vi "Client_largefile.vi"() -> ()   [LabVIEW 2016, in "Sending_larger_data.lvlib"]
uses:
  Sending_larger_data.lvlib
  <vilib>/addons/zeromq/socket_type.ctl
  <vilib>/addons/zeromq/zmq_context.lvclass
  <vilib>/addons/zeromq/zeromq.lvlib
  <vilib>/addons/zeromq/zmq_socket.lvclass
panel:
  out "Power Spectrum":dbl[](graph)
  in  "cycles":dbl=500.0 format="%#_13g"
  in  "samples":i32=5000
  in  "Send":bool
  out "reply":string[](array[string])
  out "loop":string
  out "attempt":i32
  in  "stop":bool
  in  "ntries":i32=20
  in  "endpoint":string="tcp://127.0.0.1:5555"
  in  "timeout":u32=100
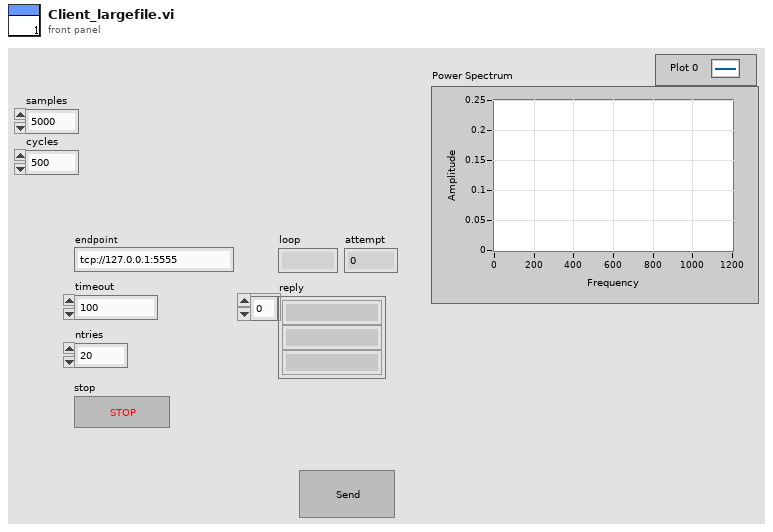
[diagram p1: front panel]
types:
  T1 = typedef "zeromq.lvlib/socket_type.ctl" = enum8{"ZMQ_PAIR", "ZMQ_PUB", "ZMQ_SUB", "ZMQ_REQ", "ZMQ_REP", "ZMQ_DEALER", "ZMQ_ROUTER", "ZMQ_PULL", "ZMQ_PUSH", "ZMQ_XPUB", "ZMQ_XSUB"}
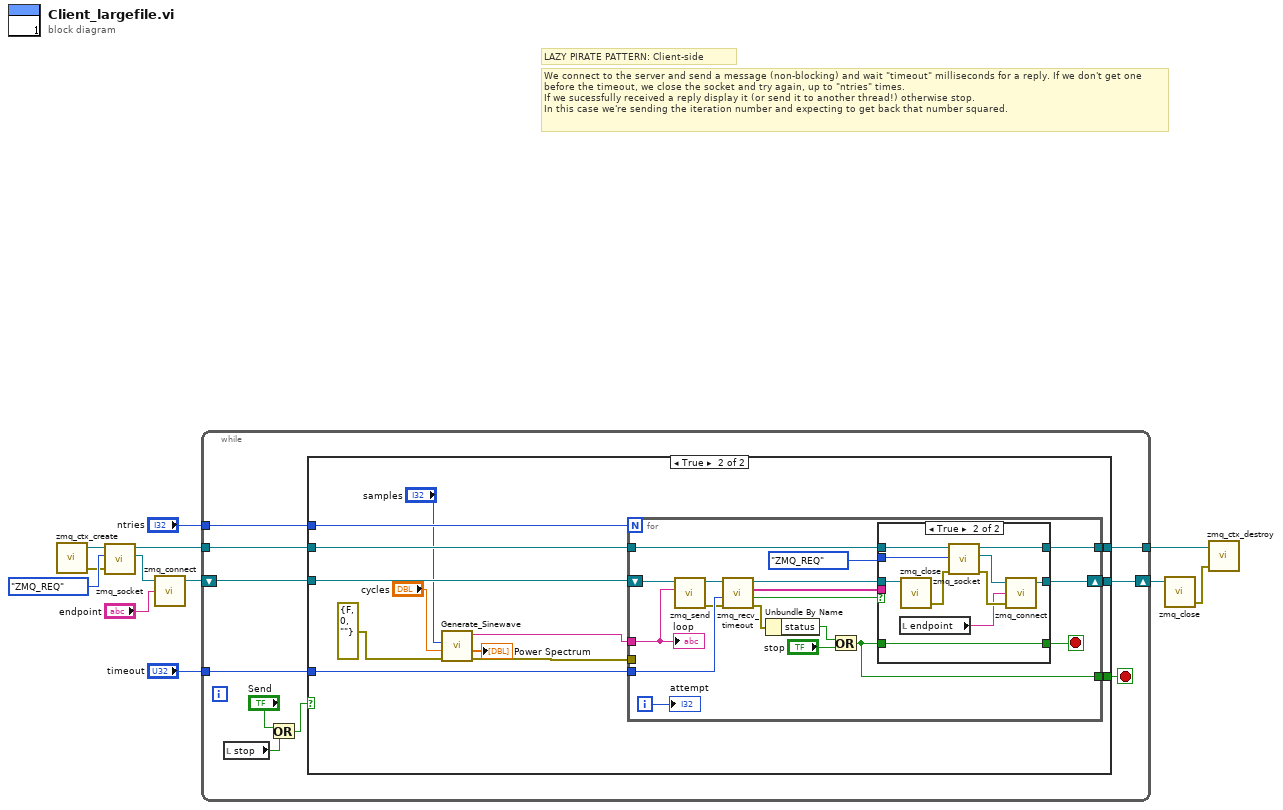
[diagram p0: block diagram]
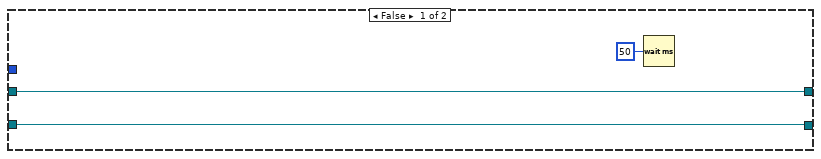
[diagram p2: hidden frame]
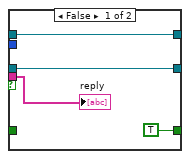
[diagram p3: hidden frame]
diagram:
  # "We connect to the server and send a message (non-blocking) and wait \"timeout\" milliseconds for a reply. If we don't get one before the timeout, we close the socket and try again, up to \"ntries\" times.\nIf we sucessfully received a reply display it (or send it to another thread!) otherwise stop.\nIn this case we're sending the iteration number and expecting to get back that number squared."
  # "LAZY PIRATE PATTERN: Client-side"
  n1 = call <vilib>:"zmq_ctx_create.vi"() -> ("error out"=w1:errorcluster, "context out"=w10:refnum<class "zmq_context.lvclass">)  [unwired: 4 in]
  n2 = call <vilib>:"zmq_socket.vi"("error in"=w1, "socket type"=socket_type."ZMQ_REQ", "context in"=w10) -> ("socket out"=w8:refnum<class "zmq_socket.lvclass">, "context out"=w7:refnum<class "zmq_context.lvclass">)  [unwired: 2 in, 1 out]
  n3 = call <vilib>:"zmq_connect.vi"("endpoint"="endpoint", "socket in"=w8) -> ("socket out"=w5:refnum<class "zmq_socket.lvclass">)  [unwired: 2 in, 1 out]
  n4 = while {
    tunnel: w7 -> [w22]
    tunnel: "timeout" -> [w21]
    tunnel: "ntries" -> [w20]
    tunnel: [w17] -> w4
    shift-right: [w16] -> w3
    shift-left: w5 -> [w18]
    stop <- w19 stop-if-true
    n5 = local read "stop"() -> (w14:bool)
    n6 = Or(x="Send", y=w14) -> (x .or. y?=w13:bool)
    n7 = case shown="True" w13 {
      tunnel: w22 -> [w24 w38]
      tunnel: w21 -> [_ w37]
      tunnel: w20 -> [_ w36]
      tunnel: [_ w35] -> w19
      tunnel: w18 -> [w25 w34]
      tunnel: [w24 w33] -> w17
      tunnel: [w25 w32] -> w16
      frame False {
        n8 = Wait (ms)(milliseconds to wait=u32 50) -> ()  [unwired: 1 out]
      }
      frame True {
        n9 = call "Generate_Sinewave.vi"("error in (no error)"=errorcluster {"status"=FALSE, "code"=0, "source"=""} ("error constant"), "cycles"="cycles", "samples"="samples") -> ("error out"=w29:errorcluster, "Power Spectrum"=→"Power Spectrum":dbl[], "Data String"=w31:string)  [unwired: 6 in]
        n10 = for {
          N: w36 -> [_]
          tunnel: w38 -> [w42]
          tunnel: w37 -> [w55]
          tunnel: w31 -> [w51]
          tunnel: [w45] -> w35
          shift-right: [w41] -> w32
          shift-left: w34 -> [w43]
          tunnel: [w40] -> w33
          tunnel: w29 -> [_]
          i -> [w50]
          stop <- w44 stop-if-true
          n11 = call <vilib>:"zmq_send.vi"("data"=w51, "socket in"=w43) -> ("error out"=w52:errorcluster, "socket out"=w53:refnum<class "zmq_socket.lvclass">)  [unwired: 5 in]
          n12 = call <vilib>:"zmq_recv_timeout.vi"("error in"=w52, "timeout (ms)"=w55, "socket in"=w53) -> ("error out"=w49:errorcluster, "timeout?"=w48:bool, "parts"=w54:string[], "socket out"=w56:refnum<class "zmq_socket.lvclass">)  [unwired: 1 in]
          n13 = Unbundle By Name(w49) -> ("status"=w47:bool)
          n14 = Or(x=w47, y="stop") -> (x .or. y?=w45:bool)
          n15 = case shown="True" w48 {
            tunnel: w56 -> [w58 w70]
            tunnel: w54 -> [w60 _]
            tunnel: w45 -> [_ w69]
            tunnel: [TRUE w69] -> w44
            tunnel: w42 -> [w57 w68]
            tunnel: [w58 w63] -> w41
            tunnel: [w57 w65] -> w40
            tunnel: socket_type."ZMQ_REQ" ("socket type") -> [_ w62]
            frame False {
              "reply" <- w60
            }
            frame True {
              n16 = local read "endpoint"() -> (w61:string)
              n17 = call <vilib>:"zmq_close.vi"("socket"=w70) -> ("error out"=w67:errorcluster)  [unwired: 4 in]
              n18 = call <vilib>:"zmq_socket.vi"("error in"=w67, "socket type"=w62, "context in"=w68) -> ("error out"=w66:errorcluster, "socket out"=w64:refnum<class "zmq_socket.lvclass">, "context out"=w65:refnum<class "zmq_context.lvclass">)  [unwired: 2 in]
              n19 = call <vilib>:"zmq_connect.vi"("error in"=w66, "endpoint"=w61, "socket in"=w64) -> ("socket out"=w63:refnum<class "zmq_socket.lvclass">)  [unwired: 1 in, 1 out]
            }
          }
          "loop" <- w51
          "attempt" <- w50
        }
      }
    }
  }
  n20 = call <vilib>:"zmq_close.vi"("socket"=w3) -> ("error out"=w2:errorcluster)  [unwired: 4 in]
  n21 = call <vilib>:"zmq_ctx_destroy.vi"("error in"=w2, "context in"=w4) -> ()  [unwired: 3 in, 1 out]
